vi "While Loop With Sweep Chart.vi"() -> ()   [LabVIEW 2012]
panel:
  in  "Knob":dbl(knob) scale=10.0..500.0
  out "While Loop Counter":dbl
  in  "Stop Button":bool
  out "Waveform Chart":dbl(graph)
  # "Frequency In Milliseconds"
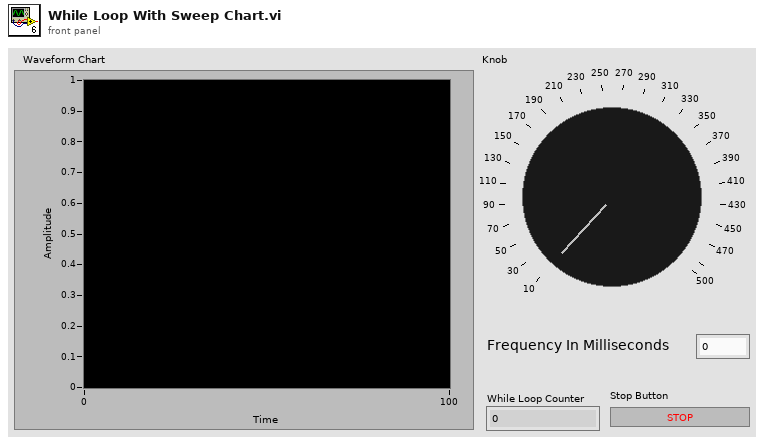
[diagram p1: front panel]
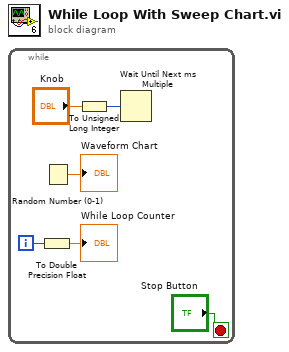
[diagram p0: block diagram]
diagram:
  n1 = while {
    i -> [w2]
    stop <- "Stop Button" stop-if-true
    n2 = To Double Precision Float(number=w2) -> (double precision float=→"While Loop Counter":dbl)
    n3 = Random Number (0-1)() -> (number: 0 to 1=→"Waveform Chart":dbl)
    n4 = To Unsigned Long Integer(number="Knob") -> (unsigned 32bit integer=w3:u32)
    n5 = Wait Until Next ms Multiple(millisecond multiple=w3) -> ()  [unwired: 1 out]
  }
